vi "DSF.Engine.Plugin.Get Inline Tx Transfer Groups.vi"(11 "Plugin in":refnum<class "DSF.Engine.Plugin.lvclass">) -> (2 "Inline Tx Transfer Groups":refnum<class "DSF.Engine.Transfer Group.lvclass">[](array[class]), 3 "Plugin out":refnum<class "DSF.Engine.Plugin.lvclass">)   [LabVIEW 2017, in "DSF.Engine.lvlib" / "DSF.Engine.Plugin.lvclass"]
uses:
  DSF.Engine.Plugin.lvclass
  Transfer/DSF.Engine.Transfer Group.lvclass
  DSF.Engine.Plugin.lvclass/DSF.Engine.Plugin.ctl
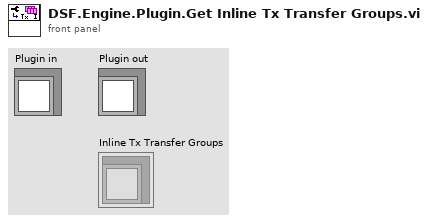
[diagram p1: front panel]
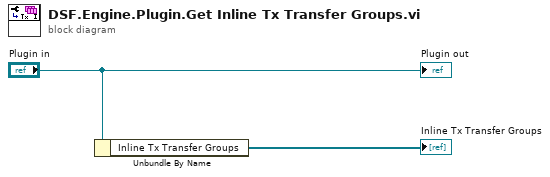
[diagram p0: block diagram]
diagram:
  n1 = Unbundle By Name("Plugin in") -> ("Inline Tx Transfer Groups"=→"Inline Tx Transfer Groups":refnum<class "DSF.Engine.Transfer Group.lvclass">[])
  "Plugin out" <- "Plugin in"
